vi "GV_Z axis.vi"() -> ()   [LabVIEW 2015]
panel:
  in  "GV_Z axis":i32
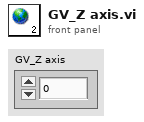
[diagram p1: front panel]
diagram:
